vi "FormulaNodeUse_Waveform_Simulator.vi"() -> ()   [LabVIEW 2017]
panel:
  out "Displacement":dbl[](array[numeric])
  in  "Amplitude":dbl
  in  "Frequency":dbl
  in  "Sampling Frequency":dbl
  in  "Number of Samples":dbl
  out "Time":dbl[](array[numeric])
  out "XY Graph":cluster{dbl[], dbl[]}(graph)
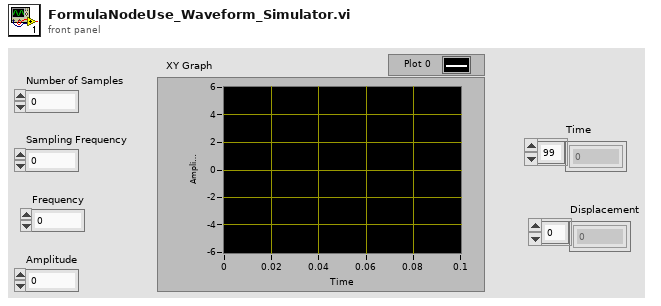
[diagram p1: front panel]
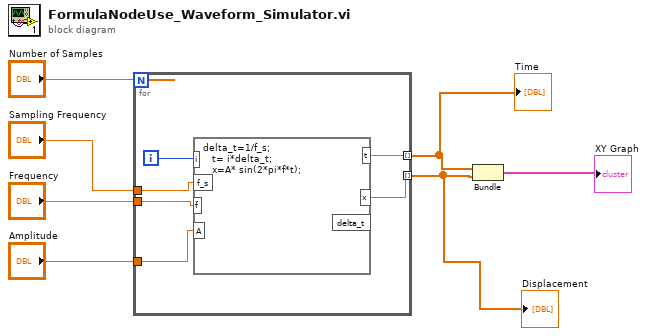
[diagram p0: block diagram]
diagram:
  n1 = for {
    N: "Number of Samples" -> [_]
    tunnel: [w12] -> w3 mode=indexing
    tunnel: "Sampling Frequency" -> [w11]
    tunnel: "Frequency" -> [w10]
    tunnel: "Amplitude" -> [w9]
    tunnel: [w8] -> w2 mode=indexing
    i -> [w13]
    n2 = formula code="delta_t=1/f_s;\n   t= i*delta_t;\n   x=A* sin(2*pi*f*t);"("i"=w13, "f_s"=w11, "f"=w10, "A"=w9) -> ("t"=w8:dbl, "x"=w12:dbl)  [unwired: 1 out]
  }
  "Time" <- w2
  "Displacement" <- w3
  n3 = Bundle(w2, w3) -> (→"XY Graph":cluster{dbl[], dbl[]})  [unwired: 1 in]
